vi "SCM4 Interlock Network Client.vi"() -> ()   [LabVIEW 2020]
doc: "Author: Scott Hannahs <sth@magnet.fsu.edu>\nCopyright 2018 Florida State University, All rights reserved."
uses:
  SCM4 Interlock LV20/RT SubVIs/RT System Auth Level.ctl
  SCM4 Interlock LV20/RT SubVIs/PS Action Control.ctl
  SubVIs/Ramp To Zero Display.ctl
  SCM4 Interlock LV20/RT SubVIs/Switch Box Status.ctl
  SubVIs/Crowbar Display.ctl
  SCM4 Interlock LV20/FPGA SubVIs/FPGA Crowbar State.ctl
  <vilib>/Utility/miscctls.llb/LVOffsetAndMultiplierTypeDef.ctl
  SCM4 Interlock LV20/RT SubVIs/Interlock RT FPGA Status Info.ctl
  SCM4 Interlock LV20/RT SubVIs/Interlock 32T FPGA Configure Parameters.ctl
  SubVIs/Interlock 32T Net Client Globals.vi
  TCP Functions/TCP Read Length and Value (STR).vi
  TCP Functions/TCP Read Length and Value (Array Str).vi
  <vilib>/Utility/miscctls.llb/LVRectTypeDef.ctl
  <vilib>/Utility/miscctls.llb/LVPointTypeDef.ctl
panel:
  in  "PS Action":T1=enum."Hold"
  in  "Clear Quench":bool
  in  "Slew rate [T/min]":dbl format="%.3g"
  out "Field [T]":dbl format="%.6f"
  in  "Setpoint [T]":dbl format="%.6g"
  out "Version":string
  in  "Clear error":bool
  in  "Front Panel Tab":T2(tab)
  out "Logic PWR V":dbl format="%.3f"
  out "Quench Loop":dbl format="%.3f"
  out "LTS Voltage":dbl format="%.3f"
  out "HTS Voltage":dbl format="%.3f"
  out "Crowbar LED":bool
  out "Close Switchbox 2":bool
  out "Crowbar Unlock Key":bool
  out "LHe Level 2":dbl format="%.1f"
  out "LHe Level 1":dbl format="%.1f"
  out "LHe Level (In)":dbl[](array[slide]) scale=0.0..60.0
  out "Crowbar Unlock Gauge":dbl(knob) scale=0.0..60.0
  out "Secondary QD Time Constant":enum16{"2000 mS", "1000 mS", "200 mS", "50 mS"}(ring)
  out "Currents":dbl[][](graph)
  out "Crowbar Latch State":T3
  out "Crowbar Fault":T4 {"Crowbar Fault" format="%02x"}
  out "Switch Box Status":T5 {"Battery Voltage" format="%.3f"; "SwBox 1 Contactor V" format="%.3f"; "SwBox 2 Contactor V" format="%.3f"; "Battery Ground V" format="%.3f"}
  out "Ramp To Zero":T6 {"Ramp To Zero Fault" format="%04x"}
  in  "Batt Mon Wait Timeout":i32=130000
  in  "Batt Mon Read Timeout":i32=10000
  in  "DAQ Iterations":u32=4096
  in  "Logic PWR Thresh":dbl format="%.1g"
  in  "Reset Battery Alarm":bool
  in  "Crowbar Unlock Safe Limit":dbl format="%.1f"
  in  "Crowbar Reset Countdown Length (ms)":i32=60000
  in  "DAQ Loop Timer (Ticks)":u32=10000
  in  "Ch Scale":dbl[](array[numeric])=[1.0, 1.0, 50.0, 20.0, 50.0, 30.0, 1.0, 200.0, 1.0, 1.0, 1.0, 1.0, 1.0] format="%.4f"
  in  "HTS DMM GPIB":u32
  in  "LTS DMM GPIB":u32
  in  "Prologix GPIB Address":string
  in  "HTS Power Supply Control":string
  in  "LTS Power Supply Control":string
  in  "Helium Level #2 VISA Resource":string
  in  "Helium Level #1 VISA Resource":string
  in  "Notification Email":string
  in  "LTS Current Mismatch":dbl format="%.1f"
  in  "HTS Current Mismatch":dbl format="%.1f"
  in  "LTS Shunt Offset (V)":dbl=40.0 format="%.4f"
  in  "Ramp To Zero Loop Time (ms)":u32=40
  in  "Client Loop Time (mS)":u32=150
  in  "Battery Low Warn":dbl format="%.1f"
  in  "Trip Threshold Currents":i16[](array[numeric])=[0, 50, 50]
  in  "SW1 Vout Thresh":dbl format="%.1g"
  in  "Quench Loop Thresh":dbl
  in  "# Low Readings":u32
  in  "Helium Low Level":dbl format="%.1f"
  in  "Crowbar Loop Time (ms)":u32=1
  in  "WDT Check Loop Ticks":u32=1000000
  in  "Contactor OFF Current":dbl format="%.1f"
  in  "Contactor ON Current":dbl format="%.1f"
  out "Start DateStamp":timestamp format="%<%H:%M:%S\n%Y/%m/%d>T"
  out "Version RT System":string
  out "Version FPGA":string
  in  "Password":string
  in  "Save FPGA Config":bool
  in  "Read FPGA Config":bool
  out "Authorized":T7
  in  "HTS Shunt Offset (V)":dbl=40.0 format="%.4f"
  out "Main Loop Ticks":u32
  out "PS Check Loop Ticks":u32
  out "DAQ Loop Ticks":u32
  out "PS Comm Time (ms)":u32
  out "DMM Comm Time (ms)":u32
  out "Watchdog Loop Ticks":u32
  out "PQD WDT Loop Ticks":u32
  out "RTZ Loop Ticks":u32
  out "Download Progress":u8(slide) scale=0.0..100.0
  in  "File List":i32(listbox)=-1
  out "Command Error":T8
  out "Comand Timing":cluster{"Command":string, "Seconds":dbl}[](array[cluster]) {"Seconds" format="%.6f"}
  out "# Clients":u32
  out "# Timeout Err":u32
  out "Chassis Temperature":fxp<+/-,16,14> format="%.2g"
  out "Status Time":dbl format="%.4f"
  out "Queue Length":i32
  out "Recorded error":errorcluster
  out "Last Batt Comm":timestamp format="%<%H:%M:%S\n%Y/%m/%d>T"
  out "Batt Alarm Text":string
  out "Error Out":errorcluster
  in  "stop":bool
  # "NHMFL 32T\nInterlock"
  # "Indicators"
  # "Helium Levels (In)"
  # "HTS Supply V"
  # "LTS Supply V"
  # "HTS LEM"
  # "HTS Shunt"
  # "LTS LEM"
  # "LTS Shunt"
  # "Quench Loop"
  # "Battery Volt 1"
  # "Battery Gnd"
  # "SW Box #1 Cont Out"
  # "SW Box #2 Cont Out"
  # "Logic Power Alarm"
  # "SW Box #1 V Out"
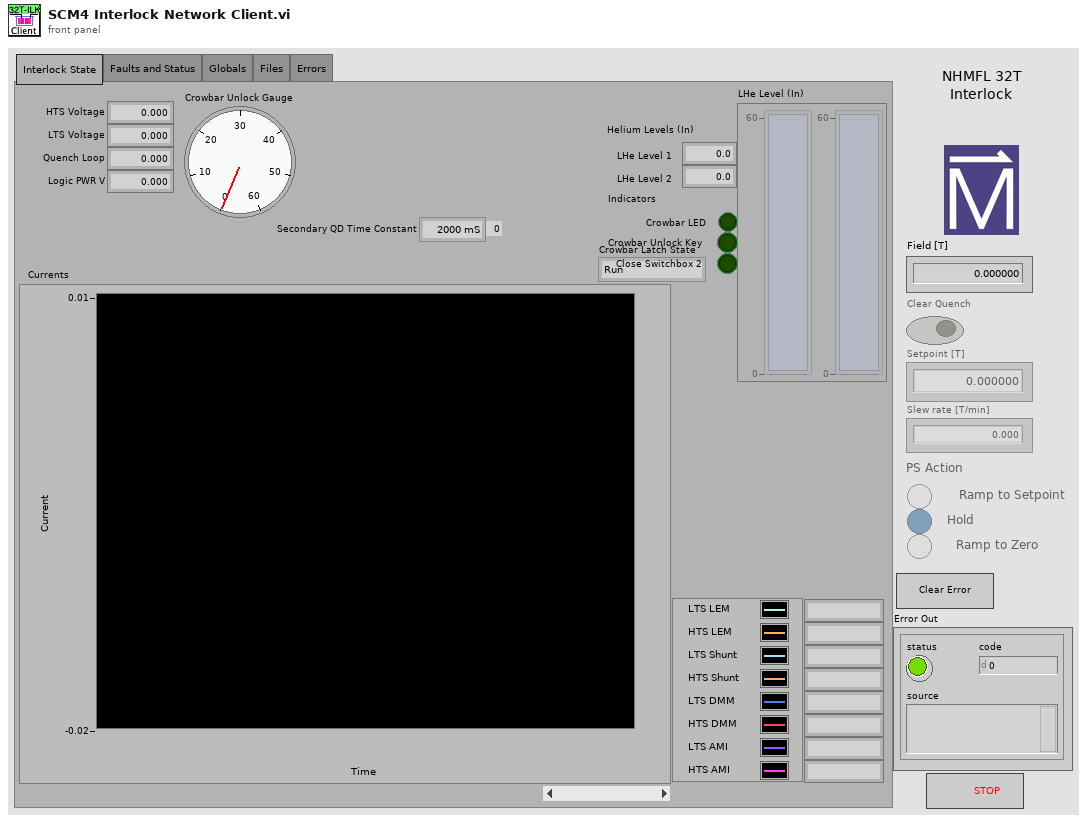
[diagram p1: front panel]
types:
  T1 = typedef "PS Action Control.ctl" = enum32{"Ramp to Setpoint", "Hold", "Ramp to Zero"}
  T2 = enum32{"Interlock State", "Faults and Status", "Globals", "Files", "Errors"}
  T3 = typedef "FPGA Crowbar State.ctl" = enum16{"Run", "Crowbar", "Reset Countdown"}
  T4 = typedef "Crowbar Display.ctl" = cluster{"Crowbar Fault":u16, "HTS LEM":bool, "LTS LEM":bool, "HTS PS Not Ready":bool, "LTS PS Not Ready":bool, "HTS Current Mismatch":bool, "LTS Current Mismatch":bool, "Quench Loop Fault":bool}
  T5 = typedef "Switch Box Status.ctl" = cluster{"Battery Voltage":dbl, "SwBox 1 Contactor V":dbl, "SwBox 2 Contactor V":dbl, "Battery Ground V":dbl}
  T6 = typedef "Ramp To Zero Display.ctl" = cluster{"Ramp To Zero Fault":u16, "Ramp to Zero Button":bool, "Protection WDT Fault":bool, "RT WDT Fault":bool, "Main WDT Fault":bool, "Ext Ramp Down WDT Fault":bool, "Crowbar WDT Fault":bool, "Logic PWR Fault":bool, "SWBox 1 V Fault":bool, "SWBox 1 Fault":bool, "SWBox 2 Fault":bool, "He Level Low":bool, "Battery Voltage Low":bool, "Battery Connect Failure":bool, "Battery Read Failure":bool, "Battery Message Failure":bool, "Battery Monitor Alarm":bool}
  T7 = typedef "RT System Auth Level.ctl" = enum16{"Read Only", "User", "Operator", "Admin"}
  T8 = cluster{"Returned String":string, "Command":string, "Option":string}
  T9 = enum8{"Enabled", "Disabled", "Disabled and Grayed Out"}
  T10 = typedef "LVPointTypeDef.ctl" = cluster{"Horizontal":i16, "Vertical":i16}
  T11 = typedef "LVRectTypeDef.ctl" = cluster{"Left":i16, "Top":i16, "Right":i16, "Bottom":i16}
  T12 = typedef "LVOffsetAndMultiplierTypeDef.ctl" = cluster{"Offset":dbl, "Multiplier":dbl}
  T13 = enum16{"Standard", "Buffered", "CRLF", "Immediate"}
  T14 = typedef "Interlock 32T FPGA Configure Parameters.ctl" = cluster{"Ch Scale":dbl[], "HTS Shunt Offset (V)":dbl, "LTS Shunt Offset (V)":dbl, "Crowbar Loop Time (ms)":u32, "Ramp To Zero Loop Time (mSec)":u32, "WDT Check Loop Ticks":u32, "Trip Threshold Currents":i16[], "Contactor OFF Current":dbl, "Contactor ON Current":dbl, "Quench Loop Thresh":dbl, "SW1 Vout Thresh":dbl, "HTS Current Mismatch":dbl, "LTS Current Mismatch":dbl, "DAQ Loop Timer (Ticks)":u32, "Crowbar Reset Countdown Length (ms)":i32, "Helium Low Levels":dbl, "# Low Readings":u32, "Battery Low Warn":dbl, "Notification Email":string, "Helium Level #1 VISA Resource":string, "Helium Level #2 VISA Resource":string, "LTS Power Supply Control":string, "HTS Power Supply Control":string, "Prologix GPIB Address":string, "LTS DMM GPIB":u32, "HTS DMM GPIB":u32, "Crowbar Unlock Safe Limit":dbl, "Logic PWR Thresh":dbl, "DAQ Iterations":i32, "Batt Mon Read Timeout":i32, "Batt Mon Wait Timeout":i32}
  T15 = typedef "Interlock RT FPGA Status Info.ctl" = cluster{"Authorized":T7, "# Clients":u32, "Chassis Temperature":fxp<+/-,16,14>, "Secondary QD Time Constant":enum16{"2000 mS", "1000 mS", "200 mS", "50 mS"}, "Crowbar Latch State":T3, "Crowbar Reset Countdown Length (ms)":i32, "Crowbar Reset Countdown":i32, "Ramp To Zero Fault":u16, "Crowbar Fault":u16, "Protection Logic V":dbl, "Quench Loop":dbl, "HTS LEM":dbl, "HTS Shunt":dbl, "LTS LEM":dbl, "LTS Shunt":dbl, "Ramp To Zero":bool, "2 Crowbar Reset Key":bool, "7 Crowbar LED":bool, "15 Close Switch Box 2 Contactor":bool, "HTS Voltage":dbl, "LTS Voltage":dbl, "DAQ Loop Ticks":u32, "PQD WDT Loop Tics":u32, "Main Loop Ticks":u32, "PS Check Loop Ticks":u32, "RTZ Loop Ticks":u32, "Watchdog Loop Ticks":u32, "LHe Level 1":dbl, "LHe Level 2":dbl, "HTS DMM":dbl, "LTS DMM":dbl, "HTS AMI430":dbl, "LTS AMI430":dbl, "Battery Monitor Alarm":bool, "Switch Box Status":T5, "PS Action":T1, "Setpoint [T]":dbl, "Field [T]":dbl, "Slew rate [T/min]":dbl, "Recorded error":errorcluster, "Last Batt Comm":timestamp, "Batt Alarm Text":string, "PS Comm Time (ms)":u32, "DMM Comm Time (ms)":u32}
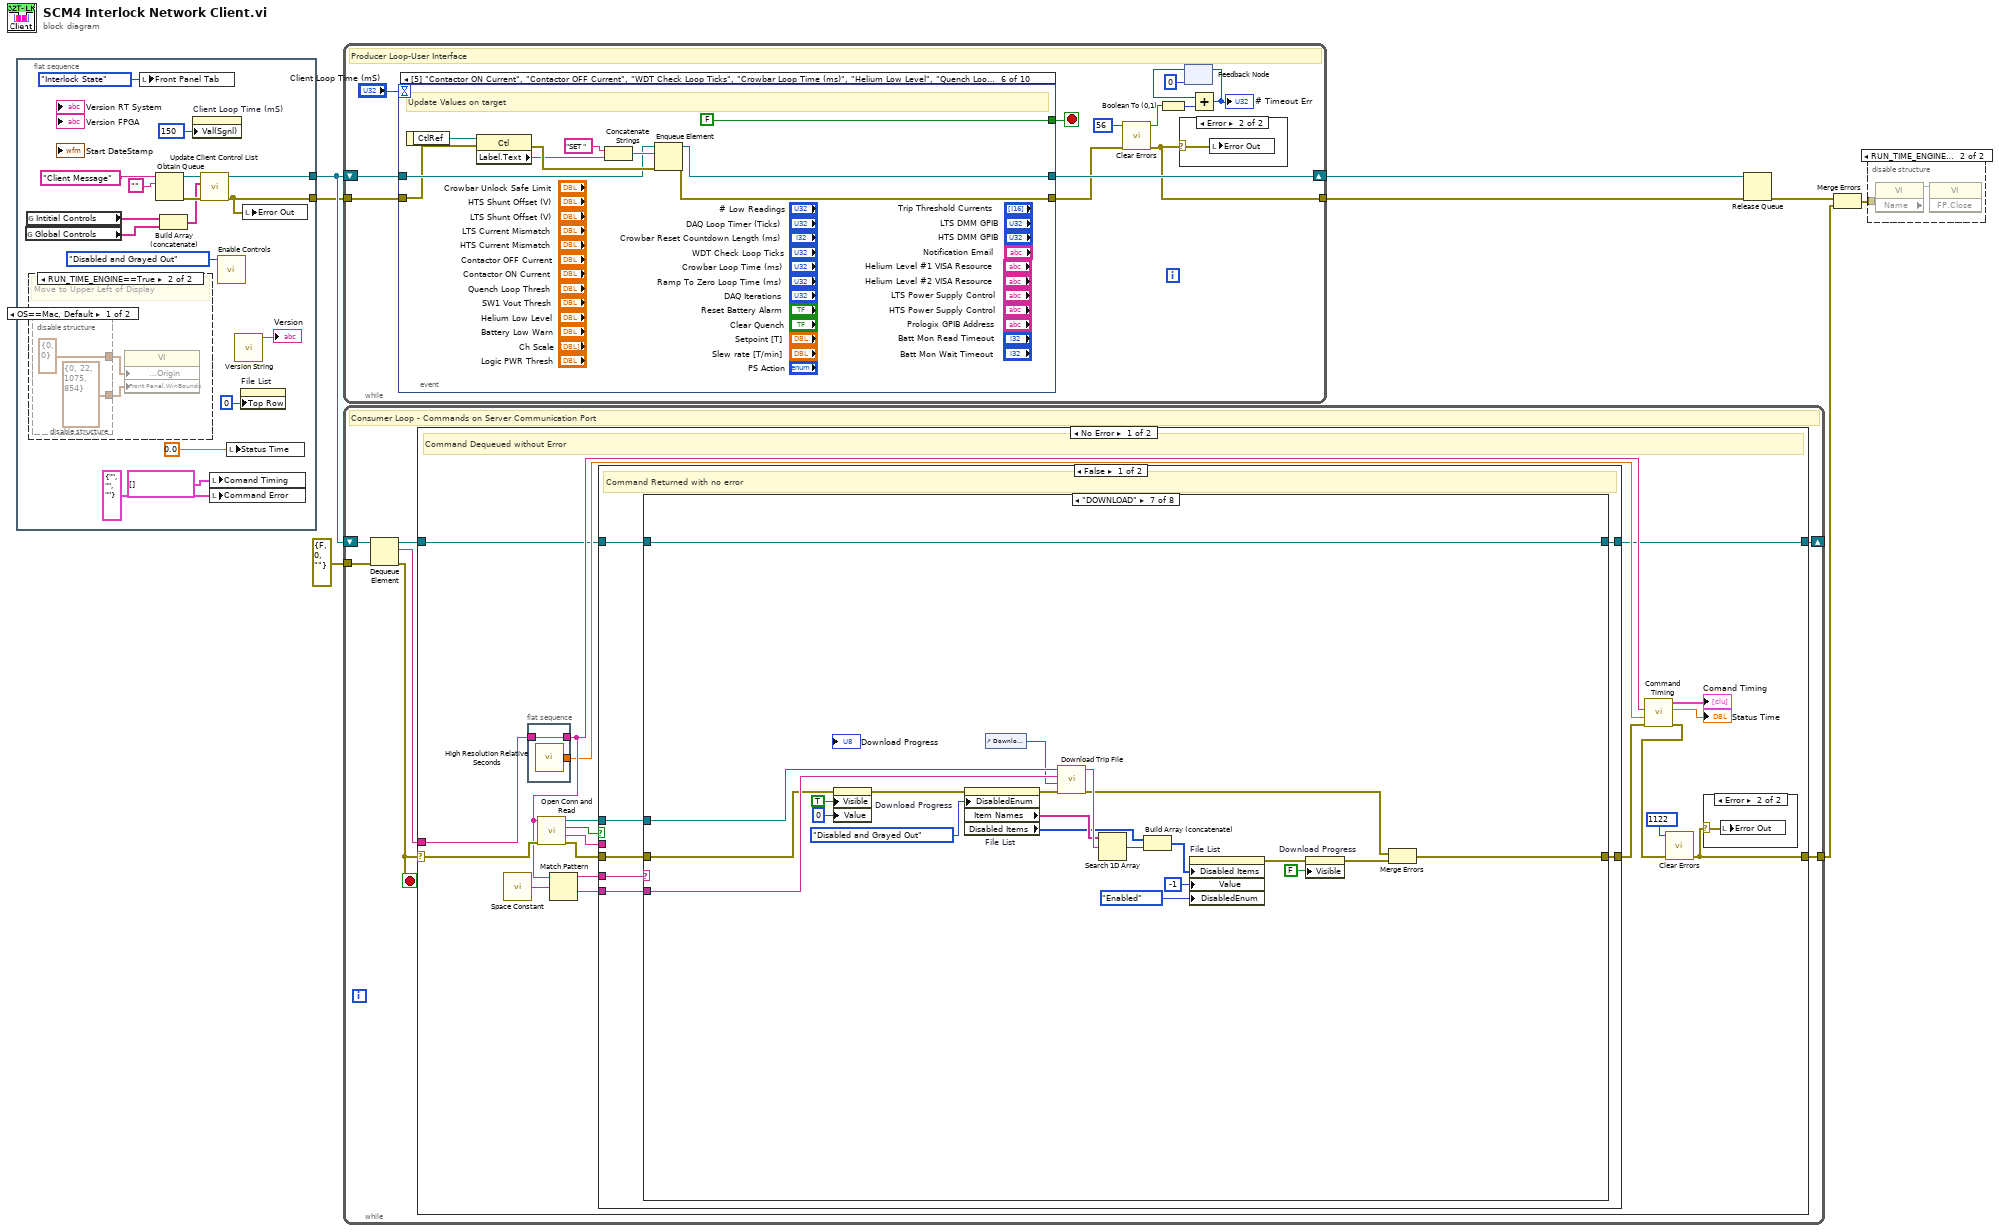
[diagram p0: block diagram]
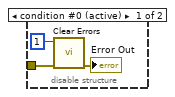
[diagram p2: hidden frame]
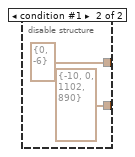
[diagram p4: hidden frame]
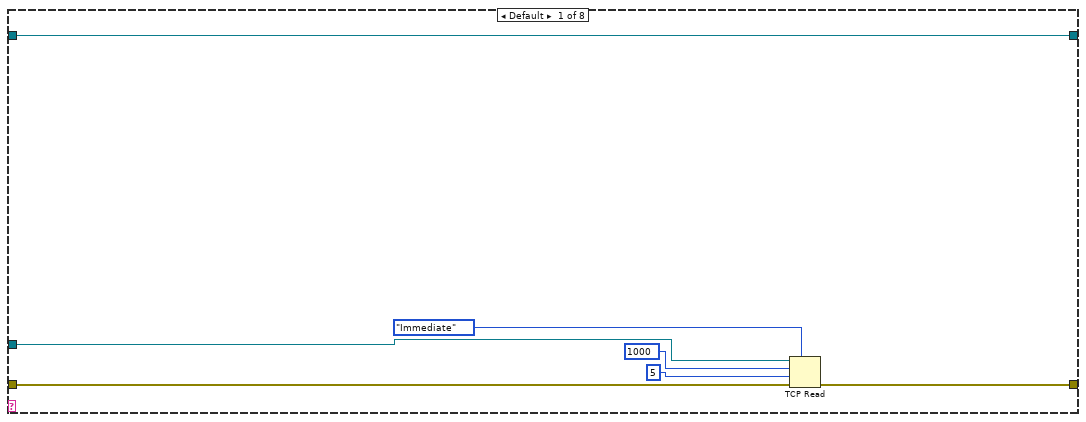
[diagram p6: hidden frame]
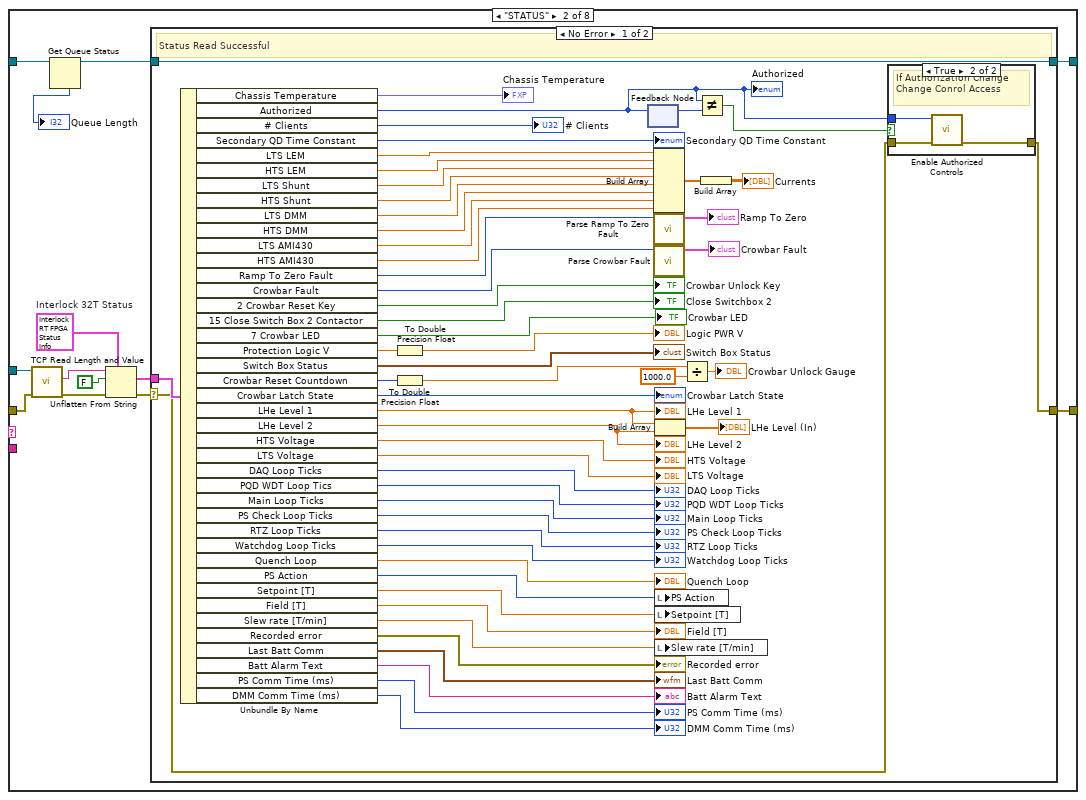
[diagram p7: hidden frame]
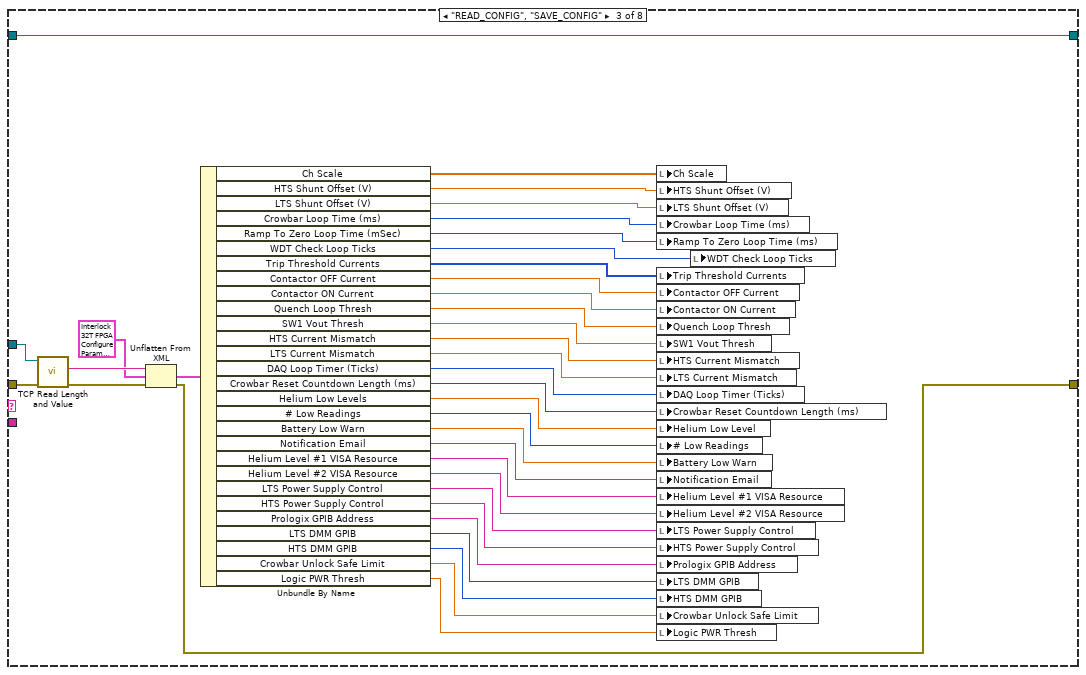
[diagram p10: hidden frame]
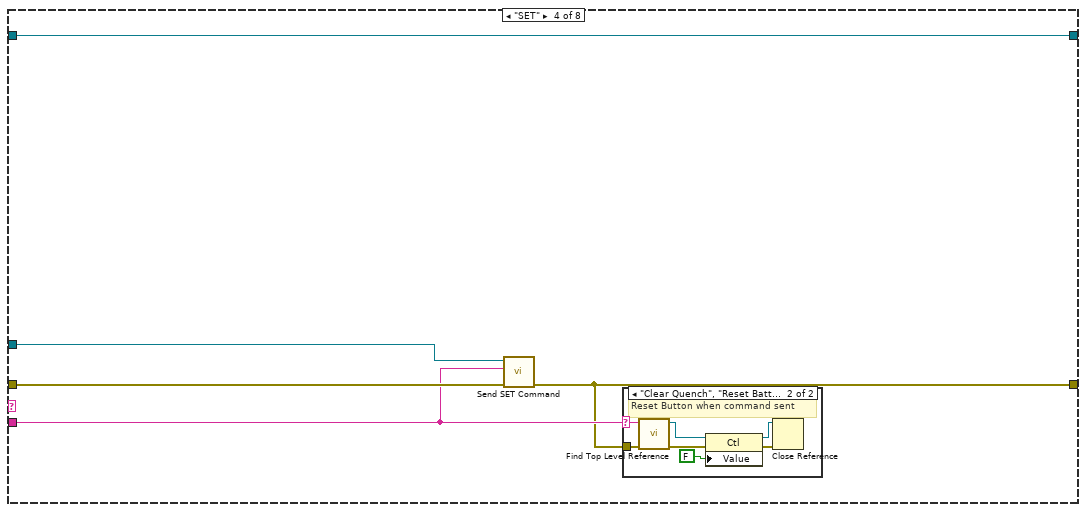
[diagram p11: hidden frame]
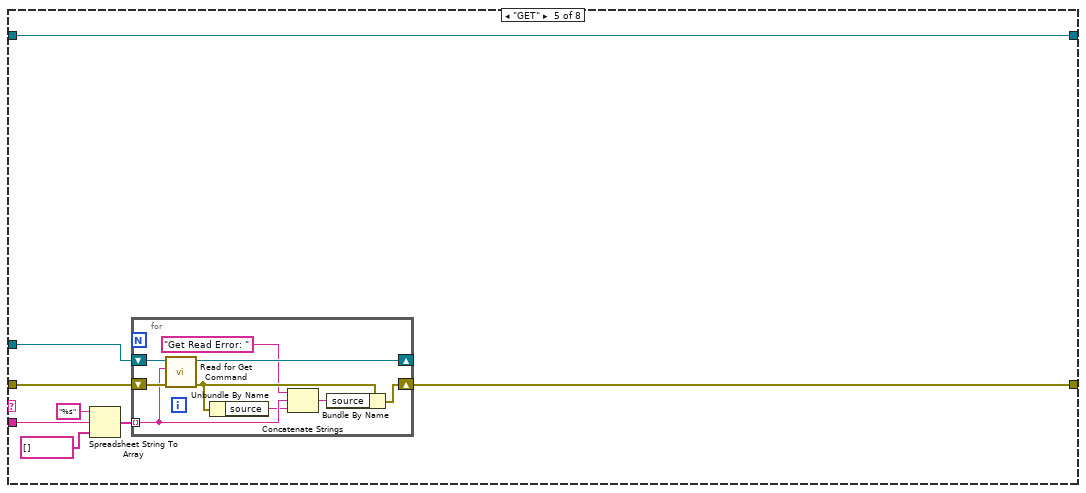
[diagram p13: hidden frame]
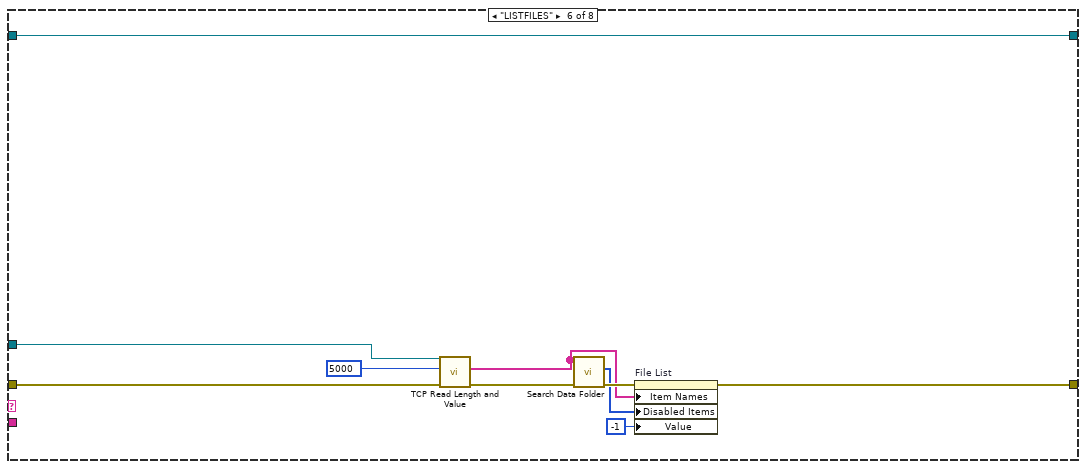
[diagram p14: hidden frame]
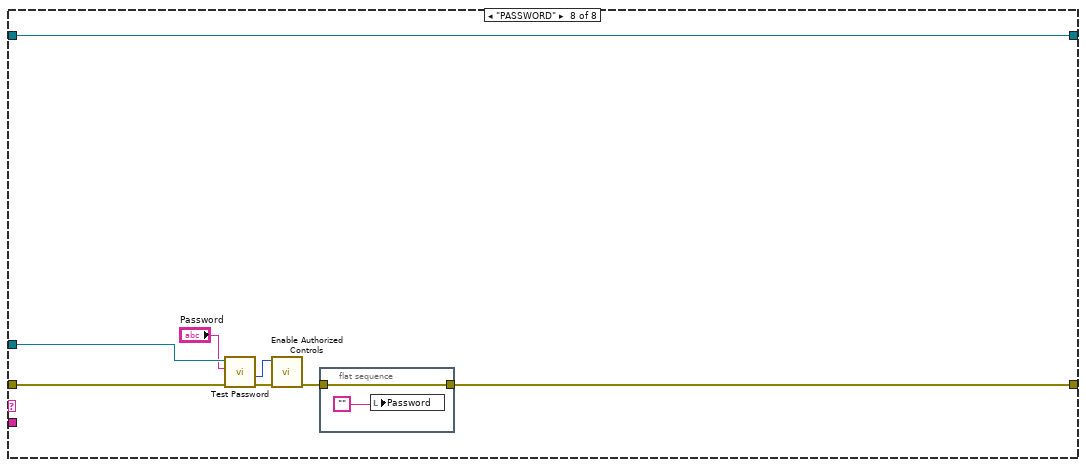
[diagram p15: hidden frame]
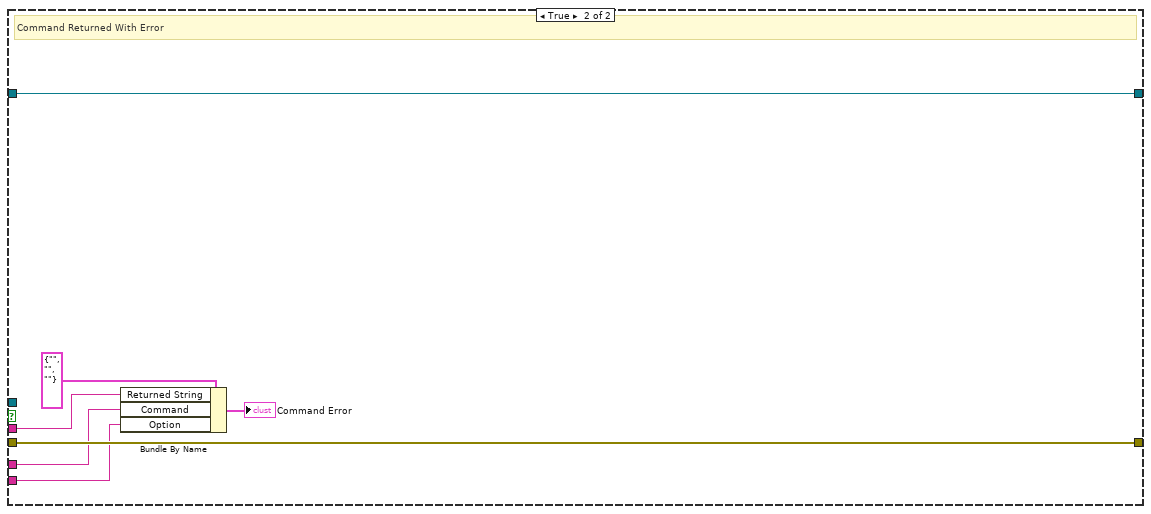
[diagram p16: hidden frame]
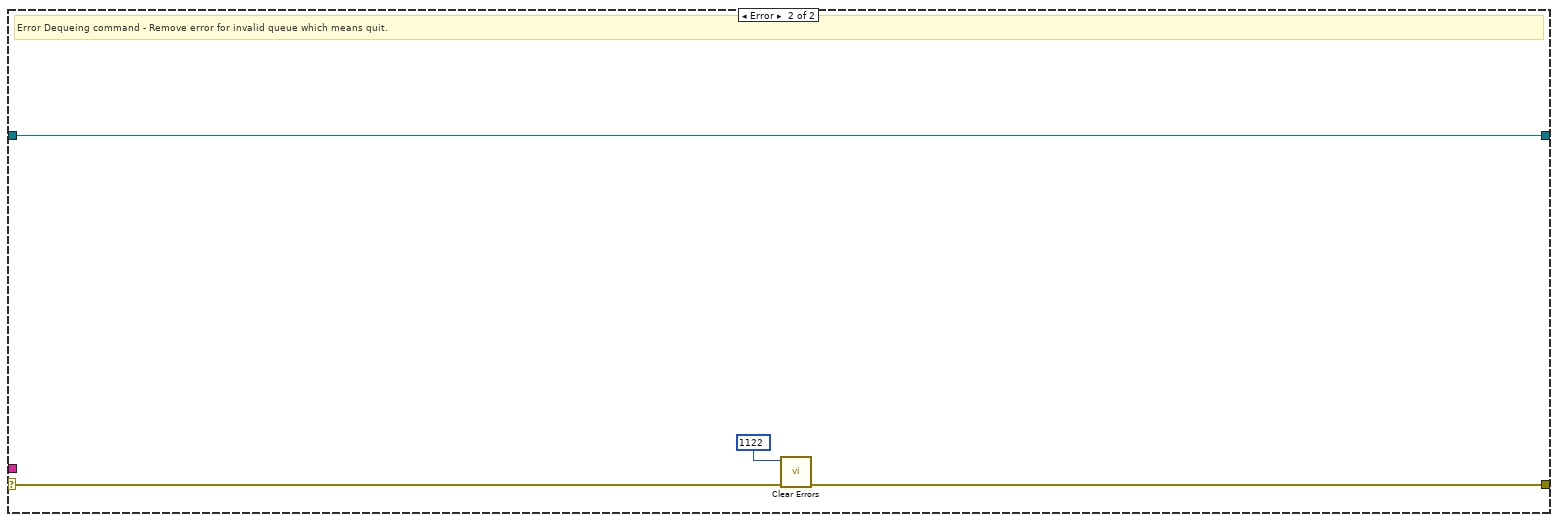
[diagram p17: hidden frame]
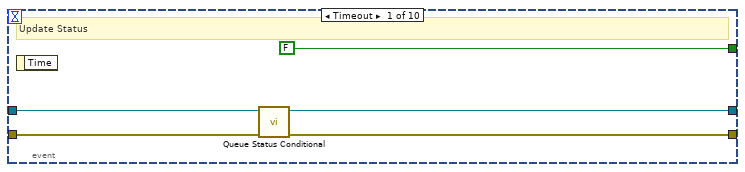
[diagram p19: hidden frame]
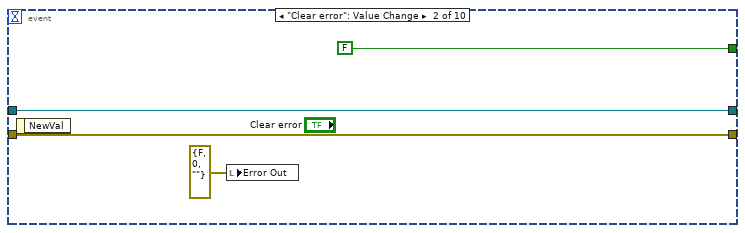
[diagram p20: hidden frame]
diagram:
  n1 = flat-sequence {
    tunnel: [w25] -> w5
    tunnel: [w20] -> w2
    frame #0 {
      n2 = global read "Interlock 32T Net Client Globals.vi" "Global Controls"() -> (w14:string[])
      n3 = global read "Interlock 32T Net Client Globals.vi" "Intitial Controls"() -> (w16:string[])
      n4 = disable-structure shown="RUN_TIME_ENGINE==True" {
        frame condition #0 (active) {
        }
        frame condition #1 {
          # "Move to Upper Left of Display"
          n5 = disable-structure shown="OS==Mac, Default" {
            disable-tunnel: [T11 {"Left"=0, "Top"=22, "Right"=1075, "Bottom"=854} ("Front Panel Window:Window Bounds") T11 {"Left"=-10, "Top"=0, "Right"=1102, "Bottom"=890} ("Front Panel Window:Window Bounds")] -> w27
            disable-tunnel: [T10 {"Horizontal"=0, "Vertical"=0} ("Front Panel Window:Origin") T10 {"Horizontal"=0, "Vertical"=-6} ("Front Panel Window:Origin")] -> w26
            frame condition #0 (active) {
            }
            frame condition #1 {
            }
          }
          n6 = property class="VI"("Front Panel Window:Origin"=w26, "Front Panel.WinBounds"=w27) -> ()  [unwired: 2 in, 2 out]
        }
      }
      n7 = local write "Front Panel Tab"(T2."Interlock State" ("Front Panel Tab")) -> ()
      n8 = Obtain Queue(name (unnamed)="Client Message", element data type="") -> (queue out=w22:refnum<queue>, error out=w21:errorcluster)  [unwired: 3 in, 1 out]
      n9 = Build Array (concatenate)(w16, w14) -> (w18:string[])
      n10 = property on="Client Loop Time (mS)" class="DigNum (strict)"("Val(Sgnl)"=u32 150 ("Value (Signaling)")) -> ()  [unwired: 2 in, 2 out]
      n11 = call "Update Client Control List.vi"("error in (no error)"=w21, "Array"=w18, "Queue in"=w22) -> ("error out"=w20:errorcluster, "Queue out"=w25:refnum<queue>)  [unwired: 6 in, 1 out]
      n12 = local write "Comand Timing"(cluster{"Command":string, "Seconds":dbl}[] [] ("Comand Timing")) -> ()
      n13 = local write "Command Error"(T8 {"Returned String"="", "Command"="", "Option"=""} ("Command Error")) -> ()
      n14 = call "Enable Controls.vi"("Enable Disable"=T9."Disabled and Grayed Out") -> ()  [unwired: 10 in, 1 out]
      n15 = local write "Status Time"(0.0 ("Field Time")) -> ()
      n16 = call "Version String.vi"() -> ("String"=→"Version":string)  [unwired: 10 in, 1 out]
      n17 = property on="File List" class="LstBox (strict)"("Top Row"=0) -> ()  [unwired: 2 in, 2 out]
      n18 = local write "Error Out"(w20) -> ()
    }
  }
  n19 = while {
    tunnel: w2 -> [w36]
    tunnel: [w37] -> w4
    shift-right: [w40] -> w7
    shift-left: w5 -> [w41]
    stop <- w38 stop-if-true
    # "Producer Loop-User Interface"
    n20 = event shown="[5] \"Contactor ON Current\", \"Contactor OFF Current\", \"WDT Check Loop Ticks\", \"Crowbar Loop Time (ms)\", \"Helium Low Level\", \"Quench Loop Thresh\", \"SW1 Vout Thresh\", \"# Low Readings\", \"Trip Threshold Currents\", \"Clear Quench\", \"HTS Shunt Offset (V)\", \"Battery Low Warn\", \"Ramp To Zero Loop Time (ms)\", \"Setpoint [T]\", \"Slew rate [T/min]\", \"PS Action\", \"HTS Current Mismatch\", \"LTS Current Mismatch\", \"LTS Shunt Offset (V)\", \"Notification Email\", \"Helium Level #1 VISA Resource\", \"Helium Level #2 VISA Resource\", \"LTS Power Supply Control\", \"HTS Power Supply Control\", \"Prologix GPIB Address\", \"LTS DMM GPIB\", \"HTS DMM GPIB\", \"Ch Scale\", \"DAQ Loop Timer (Ticks)\", \"Crowbar Reset Countdown Length (ms)\", \"Crowbar Unlock Safe Limit\", \"Reset Battery Alarm\", \"Logic PWR Thresh\", \"DAQ Iterations\": Value Change" {
      selector: _ -> [_ _ _ _ _ _ _ _ _ _]
      dyn-events: _ -> [_ _ _ _ _ _ _ _ _ _]
      timeout: "Client Loop Time (mS)" -> [_ _ _ _ _ _ _ _ _ _]
      tunnel: w36 -> [w47 w52 w67 w70 w75 w93 w103 w109 w119 w126]
      tunnel: [w46 w52 w67 w70 w74 w91 w102 w108 w113 w125] -> w39
      tunnel: [w48 w53 w66 w69 w73 w90 w101 w107 w112 w124] -> w40
      tunnel: w41 -> [w50 w53 w66 w69 w72 w94 w104 w110 w115 w127]
      tunnel: [FALSE ("NewVal") FALSE ("NewVal") FALSE ("NewVal") w68 FALSE ("NewVal") FALSE ("NewVal") FALSE ("NewVal") FALSE ("NewVal") FALSE ("NewVal") FALSE ("NewVal")] -> w38
      event Timeout {
        # "Update Status"
        n21 = event-data() -> ()  [unwired: 1 in, 1 out]
        n22 = call "Queue Status Conditional.vi"("error in (no error)"=w47, "Queue in"=w50) -> ("error out"=w46:errorcluster, "Queue out"=w48:refnum<queue>)  [unwired: 8 in]
      }
      event "Clear error": Value Change {
        n23 = event-data() -> ()  [unwired: 1 in, 1 out]
        n24 = local write "Error Out"(errorcluster {"status"=FALSE, "code"=0, "source"=""} ("Error Out")) -> ()
      }
      event "Client Loop Time (mS)": Value Change {
        w59 = 120.0  # 2 minute Display
        n25 = event-data() -> ("NewVal"=w62:u32)  [unwired: 1 in]
        n26 = Get Date/Time In Seconds() -> (seconds since 1Jan1904=w64:timestamp)
        n27 = To Double Precision Float(number=w64) -> (double precision float=w57:dbl)
        n28 = Divide(x=w62, y=1000.0) -> (x/y=w61:dbl)
        n29 = Bundle By Name(cluster=T12 {"Offset"=0.0, "Multiplier"=0.0} ("X Scale.Offset and Multiplier"), "Offset"=w57, "Multiplier"=w61) -> (w63:T12)
        n30 = Add(x=w59, y=w57) -> (x+y=w58:dbl)
        n31 = property on="Currents" class="WFChart (strict)"("XScale.Ofst&Mult"=w63, "History Data"=dbl[][] [], "XScale.Maximum"=w58, "XScale.Minimum"=w57) -> ()  [unwired: 2 in, 2 out]
      }
      event "stop": Value Change {
        n32 = event-data() -> ("NewVal"=w68:bool)  [unwired: 1 in]
      }
      event "Front Panel Tab": Value Change {
        # "Change Tab and initialize Values"
        n33 = event-data() -> ("NewVal"=w76:T2)  [unwired: 1 in]
        n34 = case shown="\"Files\"" w76 {
          tunnel: w75 -> [w77 w83 w85]
          tunnel: [w77 w82 w87] -> w74
          tunnel: [w78 w81 w88] -> w73
          tunnel: w72 -> [w78 w80 w86]
          frame "Errors", Default {
          }
          frame "Globals" {
            n35 = global read "Interlock 32T Net Client Globals.vi" "Global Controls"() -> (w79:string[])
            n36 = call "Update Client Control List.vi"("error in (no error)"=w83, "Array"=w79, "Queue in"=w80) -> ("error out"=w82:errorcluster, "Queue out"=w81:refnum<queue>)  [unwired: 6 in, 1 out]
          }
          frame "Files" {
            n37 = Enqueue Element(queue=w86, element="ListFiles", error in (no error)=w85) -> (queue out=w88:refnum<queue>, error out=w87:errorcluster)  [unwired: 1 in, 1 out]
          }
        }
      }
      event "Contactor ON Current", "Contactor OFF Current", "WDT Check Loop Ticks", "Crowbar Loop Time (ms)", "Helium Low Level", "Quench Loop Thresh", "SW1 Vout Thresh", "# Low Readings", "Trip Threshold Currents", "Clear Quench", "HTS Shunt Offset (V)", "Battery Low Warn", "Ramp To Zero Loop Time (ms)", "Setpoint [T]", "Slew rate [T/min]", "HTS Current Mismatch", "LTS Current Mismatch", "LTS Shunt Offset (V)", "Notification Email", "Helium Level #1 VISA Resource", "Helium Level #2 VISA Resource", "LTS Power Supply Control", "HTS Power Supply Control", "Prologix GPIB Address", "LTS DMM GPIB", "HTS DMM GPIB", "Ch Scale", "DAQ Loop Timer (Ticks)", "Crowbar Reset Countdown Length (ms)", "Crowbar Unlock Safe Limit", "Reset Battery Alarm", "Logic PWR Thresh", "DAQ Iterations": Value Change {
        # "Update Values on target"
        n38 = event-data() -> ("CtlRef"=w98:refnum<vi>)  [unwired: 1 in]
        n39 = property class="Ctl"(reference=w98, error in=w93) -> (error out=w96:errorcluster, "Label.Text"=w92:string)  [unwired: 1 out]
        n40 = Concatenate Strings("SET " ("string"), w92) -> (w95:string)
        n41 = Enqueue Element(queue=w94, element=w95, error in (no error)=w96) -> (queue out=w90:refnum<queue>, error out=w91:errorcluster)  [unwired: 1 in, 1 out]
      }
      event "Read FPGA Config": Value Change {
        n42 = event-data() -> ()  [unwired: 1 in, 1 out]
        n43 = Enqueue Element(queue=w104, element="Read_Config", error in (no error)=w103) -> (queue out=w101:refnum<queue>, error out=w102:errorcluster)  [unwired: 1 in, 1 out]
      }
      event "Save FPGA Config": Value Change {
        n44 = event-data() -> ()  [unwired: 1 in, 1 out]
        n45 = Enqueue Element(queue=w110, element="Save_Config", error in (no error)=w109) -> (queue out=w107:refnum<queue>, error out=w108:errorcluster)  [unwired: 1 in, 1 out]
      }
      event "File List": Value Change {
        n46 = event-data() -> ("NewVal"=w121:i32)  [unwired: 1 in]
        n47 = property on="File List" class="LstBox (strict)"(error in=w119) -> (error out=w114:errorcluster, "Item Names"=w120:string[])  [unwired: 1 in, 1 out]
        n48 = Index Array(array=w120, index=w121) -> (element=w118:string)
        n49 = Concatenate Strings("DOWNLOAD " ("string"), w118) -> (w116:string)
        n50 = Enqueue Element(queue=w115, element=w116, error in (no error)=w114) -> (queue out=w112:refnum<queue>, error out=w113:errorcluster)  [unwired: 1 in, 1 out]
      }
      event "Password": Value Change {
        n51 = event-data() -> ()  [unwired: 1 in, 6 out]
        n52 = Enqueue Element(queue=w127, element="PASSWORD" ("string"), error in (no error)=w126) -> (queue out=w124:refnum<queue>, error out=w125:errorcluster)  [unwired: 1 in, 1 out]
      }
    }
    n53 = call <vilib>:"Clear Errors.vi"("error in (no error)"=w39, "specific error code to clear (0: all)"=56) -> ("error out"=w37:errorcluster, "specific error cleared?"=w42:bool)  [unwired: 4 in]
    n54 = Boolean To (0,1)(Boolean=w42) -> (0, 1=w43:i16)
    n55 = case shown="Error" w37 {
      selector: w37 -> [_ w45]
      frame No Error {
      }
      frame Error {
        n56 = local write "Error Out"(w45) -> ()
      }
    }
    n57 = feedback #1(u32 0) -> (w33:u32)
    n58 = Add(x=w33, y=w43) -> (x+y=w34:u32)
    "# Timeout Err" <- w34
    n59 = feedback-in #1(w34) -> ()
  }
  n60 = while {
    shift-right: [w128] -> _
    shift-left: w5 -> [w130]
    tunnel: errorcluster {"status"=FALSE, "code"=0, "source"=""} ("error IO") -> [w134]
    tunnel: [w131] -> w3
    stop <- w132 stop-if-true
    # "Consumer Loop - Commands on Server Communication Port"
    n61 = Dequeue Element(queue=w130, error in (no error)=w134) -> (queue out=w129:refnum<queue>, element=w133:string, error out=w132:errorcluster)  [unwired: 1 in, 1 out]
    n62 = case shown="No Error" w132 {
      selector: w132 -> [w146 w363]
      tunnel: [w144 w362] -> w131
      tunnel: w133 -> [w143 _]
      tunnel: w129 -> [w136 w360]
      tunnel: [w135 w360] -> w128
      frame No Error {
        # "Command Dequeued without Error"
        n63 = call <vilib>:"Space Constant.vi"() -> ("String"=w148:string)
        n64 = flat-sequence {
          tunnel: [w155] -> w142
          tunnel: w143 -> [w155]
          tunnel: [w154] -> w138
          frame #0 {
            n65 = call <vilib>:"High Resolution Relative Seconds.vi"() -> ("relative seconds"=w154:dbl)
          }
        }
        n66 = call "Open Conn and Read.vi"("error in (no error)"=w146, "String"=w142) -> ("error out"=w151:errorcluster, "Returned String"=w153:string, "Returned Error"=w150:bool, "TCP Network Connection out"=w152:refnum<k5>)  [unwired: 6 in]
        n67 = Match Pattern(string=w142, regular expression=w148) -> (before substring=w149:string, after substring=w147:string)  [unwired: 1 in, 2 out]
        n68 = case shown="False" w150 {
          tunnel: [w163 w359] -> w140
          tunnel: w153 -> [_ w356]
          tunnel: w152 -> [w162 _]
          tunnel: w151 -> [w161 w359]
          tunnel: w149 -> [w160 w357]
          tunnel: w147 -> [w159 w358]
          tunnel: w136 -> [w158 w353]
          tunnel: [w157 w353] -> w135
          frame False {
            # "Command Returned with no error"
            n69 = case shown="\"DOWNLOAD\"" w160 {
              tunnel: [w165 w175 w276 w283 w299 w314 w325 w347] -> w163
              tunnel: w161 -> [w167 w182 w280 w286 w300 w320 w332 w350]
              tunnel: w162 -> [w166 w181 w281 w285 w301 w319 w342 w349]
              tunnel: w159 -> [_ _ _ w284 w298 _ w337 _]
              tunnel: w158 -> [w164 w174 w246 w282 w297 w311 w321 w343]
              tunnel: [w164 w173 w246 w282 w297 w311 w321 w343] -> w157
              frame Default {
                n70 = TCP Read(connection ID=w166, bytes to read=1000, error in (no error)=w167, 7:T13."Immediate" ("mode (standard)"), 9:5 ("timeout ms (25000)")) -> (error out=w165:errorcluster)  [unwired: 2 out]
              }
              frame "STATUS" {
                w177 = T15 {"Authorized"=enum."Read Only", "# Clients"=0, "Chassis Temperature"=0.0, "Secondary QD Time Constant"=enum."2000 mS", "Crowbar Latch State"=enum."Run", "Crowbar Reset Countdown Length (ms)"=0, "Crowbar Reset Countdown"=0, "Ramp To Zero Fault"=0, "Crowbar Fault"=0, "Protection Logic V"=0.0, "Quench Loop"=0.0, "HTS LEM"=0.0, "HTS Shunt"=0.0, "LTS LEM"=0.0, "LTS Shunt"=0.0, "Ramp To Zero"=FALSE, "2 Crowbar Reset Key"=FALSE, "7 Crowbar LED"=FALSE, "15 Close Switch Box 2 Contactor"=FALSE, "HTS Voltage"=0.0, "LTS Voltage"=0.0, "DAQ Loop Ticks"=0, "PQD WDT Loop Tics"=0, "Main Loop Ticks"=0, "PS Check Loop Ticks"=0, "RTZ Loop Ticks"=0, "Watchdog Loop Ticks"=0, "LHe Level 1"=2.148782730102539, "LHe Level 2"=3.334085464477539, "HTS DMM"=0.0, "LTS DMM"=0.0, "HTS AMI430"=0.0, "LTS AMI430"=0.0, "Battery Monitor Alarm"=FALSE, "Switch Box Status"={"Battery Voltage"=0.0, "SwBox 1 Contactor V"=0.0, "SwBox 2 Contactor V"=0.0, "Battery Ground V"=0.0}, "PS Action"=enum."Ramp to Zero", "Setpoint [T]"=0.0, "Field [T]"=0.0, "Slew rate [T/min]"=0.01, "Recorded error"={"status"=FALSE, "code"=0, "source"=""}, "Last Batt Comm"=timestamp(0 s since 1904-01-01), "Batt Alarm Text"="", "PS Comm Time (ms)"=0, "DMM Comm Time (ms)"=0}  # Interlock 32T Status
                n71 = call-poly "TCP Read Length and Value.vi"("error in (no error)"=w182, "TCP Network Connection in"=w181) -> ("error out"=w183:errorcluster, "Output"=w179:string)  [unwired: 7 in, 1 out]
                n72 = Get Queue Status(queue=w174) -> (queue out=w172:refnum<queue>, # elements in queue=→"Queue Length":i32)  [unwired: 2 in, 6 out]
                n73 = Unflatten From String(type=w177, binary string=w179, data includes array or string size? (T)=FALSE, error in (no error)=w183) -> (value=w180:T15, error out=w176:errorcluster)  [unwired: 1 in, 1 out]
                n74 = case shown="No Error" w176 {
                  selector: w176 -> [w234 w245]
                  tunnel: w180 -> [w239 _]
                  tunnel: [w233 w245] -> w175
                  tunnel: w172 -> [w197 w244]
                  tunnel: [w197 w244] -> w173
                  frame No Error {
                    # "Status Read Successful"
                    n75 = Unbundle By Name(w239) -> ("Chassis Temperature"=→"Chassis Temperature":fxp<+/-,16,14>, "Authorized"=w235:T7, "# Clients"=→"# Clients":u32, "Secondary QD Time Constant"=→"Secondary QD Time Constant":enum16{"2000 mS", "1000 mS", "200 mS", "50 mS"}, "LTS LEM"=w215:dbl, "HTS LEM"=w220:dbl, "LTS Shunt"=w219:dbl, "HTS Shunt"=w218:dbl, "LTS DMM"=w214:dbl, "HTS DMM"=w213:dbl, "LTS AMI430"=w212:dbl, "HTS AMI430"=w211:dbl, "Ramp To Zero Fault"=w210:u16, "Crowbar Fault"=w200:u16, "2 Crowbar Reset Key"=→"Crowbar Unlock Key":bool, "15 Close Switch Box 2 Contactor"=→"Close Switchbox 2":bool, "7 Crowbar LED"=→"Crowbar LED":bool, "Protection Logic V"=w206:dbl, "Switch Box Status"=→"Switch Box Status":T5, "Crowbar Reset Countdown"=w228:i32, "Crowbar Latch State"=→"Crowbar Latch State":T3, "LHe Level 1"=w223:dbl, "LHe Level 2"=w222:dbl, "HTS Voltage"=→"HTS Voltage":dbl, "LTS Voltage"=→"LTS Voltage":dbl, "DAQ Loop Ticks"=→"DAQ Loop Ticks":u32, "PQD WDT Loop Tics"=→"PQD WDT Loop Ticks":u32, "Main Loop Ticks"=→"Main Loop Ticks":u32, "PS Check Loop Ticks"=→"PS Check Loop Ticks":u32, "RTZ Loop Ticks"=→"RTZ Loop Ticks":u32, "Watchdog Loop Ticks"=→"Watchdog Loop Ticks":u32, "Quench Loop"=→"Quench Loop":dbl, "PS Action"=w204:T1, "Setpoint [T]"=w203:dbl, "Field [T]"=→"Field [T]":dbl, "Slew rate [T/min]"=w201:dbl, "Recorded error"=→"Recorded error":errorcluster, "Last Batt Comm"=→"Last Batt Comm":timestamp, "Batt Alarm Text"=→"Batt Alarm Text":string, "PS Comm Time (ms)"=→"PS Comm Time (ms)":u32, "DMM Comm Time (ms)"=→"DMM Comm Time (ms)":u32)
                    "Authorized" <- w235
                    "LHe Level 1" <- w223
                    "LHe Level 2" <- w222
                    n76 = To Double Precision Float(number=w206) -> (double precision float=→"Logic PWR V":dbl)
                    n77 = To Double Precision Float(number=w228) -> (double precision float=w190:dbl)
                    n78 = feedback-in #2(w235) -> ()
                    n79 = feedback #2() -> (w237:T7)  [unwired: 1 in]
                    n80 = Build Array(w215, w220, w219, w218, w214, w213, w212, w211) -> (w225:dbl[])
                    n81 = call "Parse Ramp To Zero Fault.vi"("Ramp To Zero Fault"=w210) -> ("Ramp To Zero"=→"Ramp To Zero":T6)  [unwired: 10 in]
                    n82 = call "Parse Crowbar Fault.vi"("Crowbar Fault"=w200) -> ("Crowbar"=→"Crowbar Fault":T4)  [unwired: 10 in]
                    n83 = Build Array(w223, w222) -> (→"LHe Level (In)":dbl[])
                    n84 = local write "PS Action"(w204) -> ()
                    n85 = local write "Setpoint [T]"(w203) -> ()
                    n86 = local write "Slew rate [T/min]"(w201) -> ()
                    n87 = Divide(x=w190, y=1000.0) -> (x/y=→"Crowbar Unlock Gauge":dbl)
                    n88 = Not Equal?(x=w235, y=w237) -> (x != y?=w236:bool)
                    n89 = Build Array(w225) -> (→"Currents":dbl[][])
                    n90 = case shown="True" w236 {
                      tunnel: w235 -> [_ w243]
                      tunnel: w234 -> [w240 w242]
                      tunnel: [w240 w241] -> w233
                      frame False {
                      }
                      frame True {
                        # "If Authorization Change\nChange Conrol Access"
                        n91 = call "Enable Authorized Controls.vi"("error in (no error)"=w242, "Authorized"=w243) -> ("error out"=w241:errorcluster)  [unwired: 9 in]
                      }
                    }
                  }
                  frame Error {
                    # "Status Not Read"
                  }
                }
              }
              frame "READ_CONFIG", "SAVE_CONFIG" {
                n92 = call-poly "TCP Read Length and Value.vi"("error in (no error)"=w280, "TCP Network Connection in"=w281) -> ("error out"=w278:errorcluster, "Output"=w279:string)  [unwired: 7 in, 1 out]
                n93 = Unflatten From XML(xml string=w279, type=T14 {"Ch Scale"=[1.0, 1.0, 50.0, 20.0, 50.0, 30.0, 1.0, 200.0, 1.0, 1.0, 1.0, 1.0, 1.0], "HTS Shunt Offset (V)"=0.999969482421875, "LTS Shunt Offset (V)"=0.0, "Crowbar Loop Time (ms)"=512, "Ramp To Zero Loop Time (mSec)"=10, "WDT Check Loop Ticks"=0, "Trip Threshold Currents"=[0, 50, 50], "Contactor OFF Current"=0.001953125, "Contactor ON Current"=16.0, "Quench Loop Thresh"=1.5, "SW1 Vout Thresh"=15.0, "HTS Current Mismatch"=1.0, "LTS Current Mismatch"=1.0, "DAQ Loop Timer (Ticks)"=0, "Crowbar Reset Countdown Length (ms)"=4000000, "Helium Low Levels"=3.0, "# Low Readings"=3, "Battery Low Warn"=450.0, "Notification Email"="NHMFL DCFF Turnover <turnover@magnet.fsu.edu>", "Helium Level #1 VISA Resource"="TCPIP0::m1700-17-190::7180::SOCKET", "Helium Level #2 VISA Resource"="TCPIP0::m1700-17-191::7180::SOCKET", "LTS Power Supply Control"="TCPIP0::146.201.236.95::7180::SOCKET", "HTS Power Supply Control"="TCPIP0::146.201.236.94::7180::SOCKET", "Prologix GPIB Address"="tcpip::prologix-00-21-69-01-04-af.ad.magnet.fsu.edu::1234::socket", "LTS DMM GPIB"=23, "HTS DMM GPIB"=25, "Crowbar Unlock Safe Limit"=0.0, "Logic PWR Thresh"=1.0, "DAQ Iterations"=4096, "Batt Mon Read Timeout"=10000, "Batt Mon Wait Timeout"=130000} ("Interlock 32T FPGA Configuration Values In"), error in (no error)=w278) -> (value=w275:T14, error out=w276:errorcluster)
                n94 = Unbundle By Name(w275) -> ("Ch Scale"=w274:dbl[], "HTS Shunt Offset (V)"=w272:dbl, "LTS Shunt Offset (V)"=w271:dbl, "Crowbar Loop Time (ms)"=w273:u32, "Ramp To Zero Loop Time (mSec)"=w268:u32, "WDT Check Loop Ticks"=w269:u32, "Trip Threshold Currents"=w270:i16[], "Contactor OFF Current"=w262:dbl, "Contactor ON Current"=w263:dbl, "Quench Loop Thresh"=w264:dbl, "SW1 Vout Thresh"=w265:dbl, "HTS Current Mismatch"=w267:dbl, "LTS Current Mismatch"=w266:dbl, "DAQ Loop Timer (Ticks)"=w251:u32, "Crowbar Reset Countdown Length (ms)"=w249:i32, "Helium Low Levels"=w250:dbl, "# Low Readings"=w261:u32, "Battery Low Warn"=w260:dbl, "Notification Email"=w259:string, "Helium Level #1 VISA Resource"=w258:string, "Helium Level #2 VISA Resource"=w257:string, "LTS Power Supply Control"=w256:string, "HTS Power Supply Control"=w255:string, "Prologix GPIB Address"=w254:string, "LTS DMM GPIB"=w253:u32, "HTS DMM GPIB"=w252:u32, "Crowbar Unlock Safe Limit"=w248:dbl, "Logic PWR Thresh"=w247:dbl)
                n95 = local write "Ch Scale"(w274) -> ()
                n96 = local write "HTS Shunt Offset (V)"(w272) -> ()
                n97 = local write "LTS Shunt Offset (V)"(w271) -> ()
                n98 = local write "Crowbar Loop Time (ms)"(w273) -> ()
                n99 = local write "Ramp To Zero Loop Time (ms)"(w268) -> ()
                n100 = local write "Trip Threshold Currents"(w270) -> ()
                n101 = local write "Contactor OFF Current"(w262) -> ()
                n102 = local write "Contactor ON Current"(w263) -> ()
                n103 = local write "Quench Loop Thresh"(w264) -> ()
                n104 = local write "SW1 Vout Thresh"(w265) -> ()
                n105 = local write "HTS Current Mismatch"(w267) -> ()
                n106 = local write "LTS Current Mismatch"(w266) -> ()
                n107 = local write "DAQ Loop Timer (Ticks)"(w251) -> ()
                n108 = local write "Crowbar Reset Countdown Length (ms)"(w249) -> ()
                n109 = local write "Helium Low Level"(w250) -> ()
                n110 = local write "# Low Readings"(w261) -> ()
                n111 = local write "Battery Low Warn"(w260) -> ()
                n112 = local write "Notification Email"(w259) -> ()
                n113 = local write "Helium Level #1 VISA Resource"(w258) -> ()
                n114 = local write "Helium Level #2 VISA Resource"(w257) -> ()
                n115 = local write "LTS Power Supply Control"(w256) -> ()
                n116 = local write "HTS Power Supply Control"(w255) -> ()
                n117 = local write "Prologix GPIB Address"(w254) -> ()
                n118 = local write "LTS DMM GPIB"(w253) -> ()
                n119 = local write "HTS DMM GPIB"(w252) -> ()
                n120 = local write "Crowbar Unlock Safe Limit"(w248) -> ()
                n121 = local write "Logic PWR Thresh"(w247) -> ()
                n122 = local write "WDT Check Loop Ticks"(w269) -> ()
              }
              frame "SET" {
                n123 = call "Send SET Command.vi"("error in (no error)"=w286, "Control Name"=w284, "TCP Network Connection in"=w285) -> ("error out"=w283:errorcluster)  [unwired: 8 in]
                n124 = case shown="\"Clear Quench\", \"Reset Battery Alarm\"" w284 {
                  selector: w284 -> [_ w293]
                  tunnel: w283 -> [_ w287]
                  frame Default {
                  }
                  frame "Clear Quench", "Reset Battery Alarm" {
                    # "Reset Button when command sent"
                    n125 = call "Find Top Level Reference.vi"("error in (no error)"=w287, "String"=w293) -> ("error out"=w288:errorcluster, "Ctl Refnum"=w292:refnum<vi>)  [unwired: 8 in]
                    n126 = property class="Ctl"(reference=w292, error in=w288, "Value"=FALSE) -> (reference out=w289:refnum<vi>, error out=w290:errorcluster)
                    n127 = Close Reference(reference=w289, error in (no error)=w290) -> ()  [unwired: 1 out]
                  }
                }
              }
              frame "GET" {
                n128 = Spreadsheet String To Array(format string="%s", spreadsheet string=w298, array type (2D Dbl)=string[] []) -> (array=w296:string[])  [unwired: 1 in]
                n129 = for {
                  tunnel: w296 -> [w305] mode=indexing
                  shift-right: [w307] -> w299
                  shift-left: w300 -> [w309]
                  shift-right: [w308] -> _
                  shift-left: w301 -> [w310]
                  n130 = call "Read for Get Command.vi"("error in (no error)"=w309, "Control Name"=w305, "TCP Network Connection in"=w310) -> ("error out"=w306:errorcluster, "TCP Network Connection out"=w308:refnum<k5>)  [unwired: 7 in]
                  n131 = Unbundle By Name(w306) -> ("source"=w304:string)
                  n132 = Concatenate Strings("Get Read Error: " ("string"), w305, w304) -> (w303:string)
                  n133 = Bundle By Name(cluster=w306, "source"=w303) -> (w307:errorcluster)
                }
              }
              frame "LISTFILES" {
                n134 = call-poly "TCP Read Length and Value.vi"("error in (no error)"=w320, "timeout ms (1000)"=5000, "TCP Network Connection in"=w319) -> ("error out"=w318:errorcluster, "Output"=w315:string[])  [unwired: 6 in, 1 out]
                n135 = call "Search Data Folder.vi"("error in (no error)"=w318, "Server File List"=w315) -> ("error out"=w317:errorcluster, "Disabled Items"=w316:i32[])  [unwired: 8 in]
                n136 = property on="File List" class="LstBox (strict)"(error in=w317, "Item Names"=w315, "Disabled Items"=w316, "Value"=-1 ("File List")) -> (error out=w314:errorcluster)  [unwired: 1 in, 1 out]
              }
              frame "DOWNLOAD" {
                n137 = property on="Download Progress" class="Slide (strict)"(error in=w332, "Visible"=TRUE, "Value"=u8 0 ("Download Progress")) -> (error out=w327:errorcluster)  [unwired: 1 in, 1 out]
                n138 = property on="File List" class="LstBox (strict)"(error in=w327, "DisabledEnum"=T9."Disabled and Grayed Out" ("Disabled")) -> (error out=w326:errorcluster, "Item Names"=w323:string[], "Disabled Items"=w322:i32[])  [unwired: 1 in, 1 out]
                n139 = control-ref of="Download Progress"() -> (w334:refnum<vi>)
                n140 = call "Download Trip File.vi"("error in (no error)"=w326, "Download Progress Ref"=w334, "File Name"=w337, "TCP Network Connection in"=w342) -> ("error out"=w324:errorcluster, "File Name Out"=w339:string)  [unwired: 6 in]
                n141 = Search 1D Array(1D array=w323, element=w339) -> (index of element=w340:i32)  [unwired: 1 in]
                n142 = Build Array (concatenate)(w322, w340) -> (w341:i32[])
                n143 = property on="File List" class="LstBox (strict)"("Disabled Items"=w341, "Value"=-1 ("File List"), "DisabledEnum"=T9."Enabled" ("Disabled")) -> (error out=w331:errorcluster)  [unwired: 2 in, 1 out]
                n144 = property on="Download Progress" class="Slide (strict)"(error in=w331, "Visible"=FALSE) -> (error out=w330:errorcluster)  [unwired: 1 in, 1 out]
                n145 = Merge Errors(w324, w330) -> (w325:errorcluster)
              }
              frame "PASSWORD" {
                n146 = call "Test Password.vi"("error in (no error)"=w350, "String"="Password", "TCP Network Connection in"=w349) -> ("error out"=w344:errorcluster, "Authorized"=w346:T7)  [unwired: 6 in, 1 out]
                n147 = call "Enable Authorized Controls.vi"("error in (no error)"=w344, "Authorized"=w346) -> ("error out"=w345:errorcluster)  [unwired: 9 in]
                n148 = flat-sequence {
                  tunnel: w345 -> [w352]
                  tunnel: [w352] -> w347
                  frame #0 {
                    n149 = local write "Password"("") -> ()
                  }
                }
              }
            }
          }
          frame True {
            # "Command Returned With Error"
            n150 = Bundle By Name(cluster=T8 {"Returned String"="", "Command"="", "Option"=""} ("Command Error"), "Returned String"=w356, "Command"=w357, "Option"=w358) -> (→"Command Error":T8)
          }
        }
        n151 = call "Command Timing.vi"("error in (no error)"=w140, "Seconds"=w138, "Command"=w142) -> ("error out"=w141:errorcluster, "Status Time"=→"Status Time":dbl, "Comand Timing out"=→"Comand Timing":cluster{"Command":string, "Seconds":dbl}[])  [unwired: 6 in]
        n152 = call <vilib>:"Clear Errors.vi"("error in (no error)"=w141, "specific error code to clear (0: all)"=1122) -> ("error out"=w144:errorcluster)  [unwired: 4 in, 1 out]
        n153 = case shown="Error" w144 {
          selector: w144 -> [_ w156]
          frame No Error {
          }
          frame Error {
            n154 = local write "Error Out"(w156) -> ()
          }
        }
      }
      frame Error {
        # "Error Dequeing command - Remove error for invalid queue which means quit."
        n155 = call <vilib>:"Clear Errors.vi"("error in (no error)"=w363, "specific error code to clear (0: all)"=1122) -> ("error out"=w362:errorcluster)  [unwired: 4 in, 1 out]
      }
    }
  }
  n156 = Release Queue(queue=w7, error in (no error)=w4) -> (error out=w6:errorcluster)  [unwired: 1 in, 2 out]
  n157 = Merge Errors(w6, w3) -> (w1:errorcluster)
  n158 = disable-structure shown="RUN_TIME_ENGINE==True" {
    disable-tunnel: w1 -> [w366 _]
    frame condition #0 (active) {
      n159 = call <vilib>:"Clear Errors.vi"("error in (no error)"=w366, "specific error code to clear (0: all)"=1) -> ("error out"=→"Error Out":errorcluster)  [unwired: 4 in, 1 out]
    }
    frame condition #1 {
      n160 = property class="VI" props=["Name"]() -> (reference out=w367:refnum<vi>)  [unwired: 2 in, 2 out]
      n161 = invoke class="VI" method="FP.Close"(reference=w367) -> ()  [unwired: 2 in, 3 out]
    }
  }
